vi "Autonomous Independent.vi"() -> ()   [LabVIEW 2016]
doc: "This VI is called when autonomous begins, and will automatically be terminated when autonomous ends. You can carry out timed or sensor driven robot movement independently without needing to return to the caller."
uses:
  2_8_17/Auto_Action.ctl
  <vilib>/Rock Robotics/WPI/Solenoid/WPI_SolenoidValue.ctl
  <vilib>/Rock Robotics/Network Tables/NT Read Number.vi
  <vilib>/Rock Robotics/WPI/Ultrasonic/WPI_SonarSRF04DigitalRefNum Registry Get.vi
  <vilib>/Rock Robotics/WPI/Ultrasonic/WPI_SonarSRF04DigitalGetRange.vi
panel:
  in  "Value":T1=enum."Forward"
  out "Auto Mode":dbl=3.0
  in  "Auton_Modes":T3(array[cluster])=[{"Actions"=[{"Effort"=0.55, "Duration"=3.5, "Action"=enum."Nothing"}, {"Effort"=0.0, "Duration"=0.0, "Action"=enum."Nothing"}]}, {"Actions"=[{"Effort"=0.0, "Duration"=1.0, "Action"=enum."Nothing"}, {"Effort"=0.75, "Duration"=5.0, "Action"=enum."Nothing"}, {"Effort"=0.0, "Duration"=1.0, "Action"=enum."Nothing"}]}, {"Actions"=[{"Effort"=1.0, "Duration"=3.0, "Action"=enum."Nothing"}, {"Effort"=0.0, "Duration"=1.0, "Action"=enum."Nothing"}, {"Effort"=0.75, "Duration"=3.5, "Action"=enum."Nothing"}, {"Effort"=0.0, "Duration"=1.0, "Action"=enum."Nothing"}]}, {"Actions"=[{"Effort"=0.0, "Duration"=0.5, "Action"=enum."Nothing"}, {"Effort"=0.8, "Duration"=5.28, "Action"=enum."Nothing"}, {"Effort"=0.0, "Duration"=1.0, "Action"=enum."Nothing"}, {"Effort"=-0.8, "Duration"=1.8, "Action"=enum."Nothing"}, {"Effort"=0.0, "Duration"=0.1, "Action"=enum."Nothing"}, {"Effort"=0.8, "Duration"=1.75, "Action"=enum."Nothing"}, {"Effort"=0.0, "Duration"=0.5, "Action"=enum."Nothing"}, {"Effort"=0.0, "Duration"=4.0, "Action"=enum."Nothing"}]}, {"Actions"=[{"Effort"=0.0, "Duration"=0.0, "Action"=enum."Nothing"}, {"Effort"=1.0, "Duration"=0.1, "Action"=enum."Nothing"}, {"Effort"=0.0, "Duration"=0.1, "Action"=enum."Nothing"}, {"Effort"=1.0, "Duration"=3.0, "Action"=enum."Nothing"}]}, {"Actions"=[{"Effort"=0.0, "Duration"=0.0, "Action"=enum."Nothing"}, {"Effort"=1.0, "Duration"=0.1, "Action"=enum."Nothing"}, {"Effort"=0.0, "Duration"=0.1, "Action"=enum."Nothing"}, {"Effort"=1.0, "Duration"=3.0, "Action"=enum."Nothing"}]}, {"Actions"=[{"Effort"=0.55, "Duration"=4.0, "Action"=enum."Nothing"}, {"Effort"=0.0, "Duration"=1.0, "Action"=enum."Nothing"}, {"Effort"=-0.5, "Duration"=0.6, "Action"=enum."Nothing"}, {"Effort"=0.75, "Duration"=1.0, "Action"=enum."Nothing"}, {"Effort"=0.0, "Duration"=1.0, "Action"=enum."Nothing"}, {"Effort"=0.75, "Duration"=3.0, "Action"=enum."Nothing"}]}, {"Actions"=[{"Effort"=0.0, "Duration"=0.5, "Action"=enum."Nothing"}, {"Effort"=0.55, "Duration"=4.25, "Action"=enum."Nothing"}, {"Effort"=0.0, "Duration"=0.0, "Action"=enum."Nothing"}, {"Effort"=0.0, "Duration"=0.3, "Action"=enum."Nothing"}, {"Effort"=0.9, "Duration"=2.0, "Action"=enum."Nothing"}]}, {"Actions"=[{"Effort"=0.0, "Duration"=0.0, "Action"=enum."Nothing"}]}]
  # "Nothing"
  # "Boiler Side Gear"
  # "Middle Gear"
  # "Farside Gear"
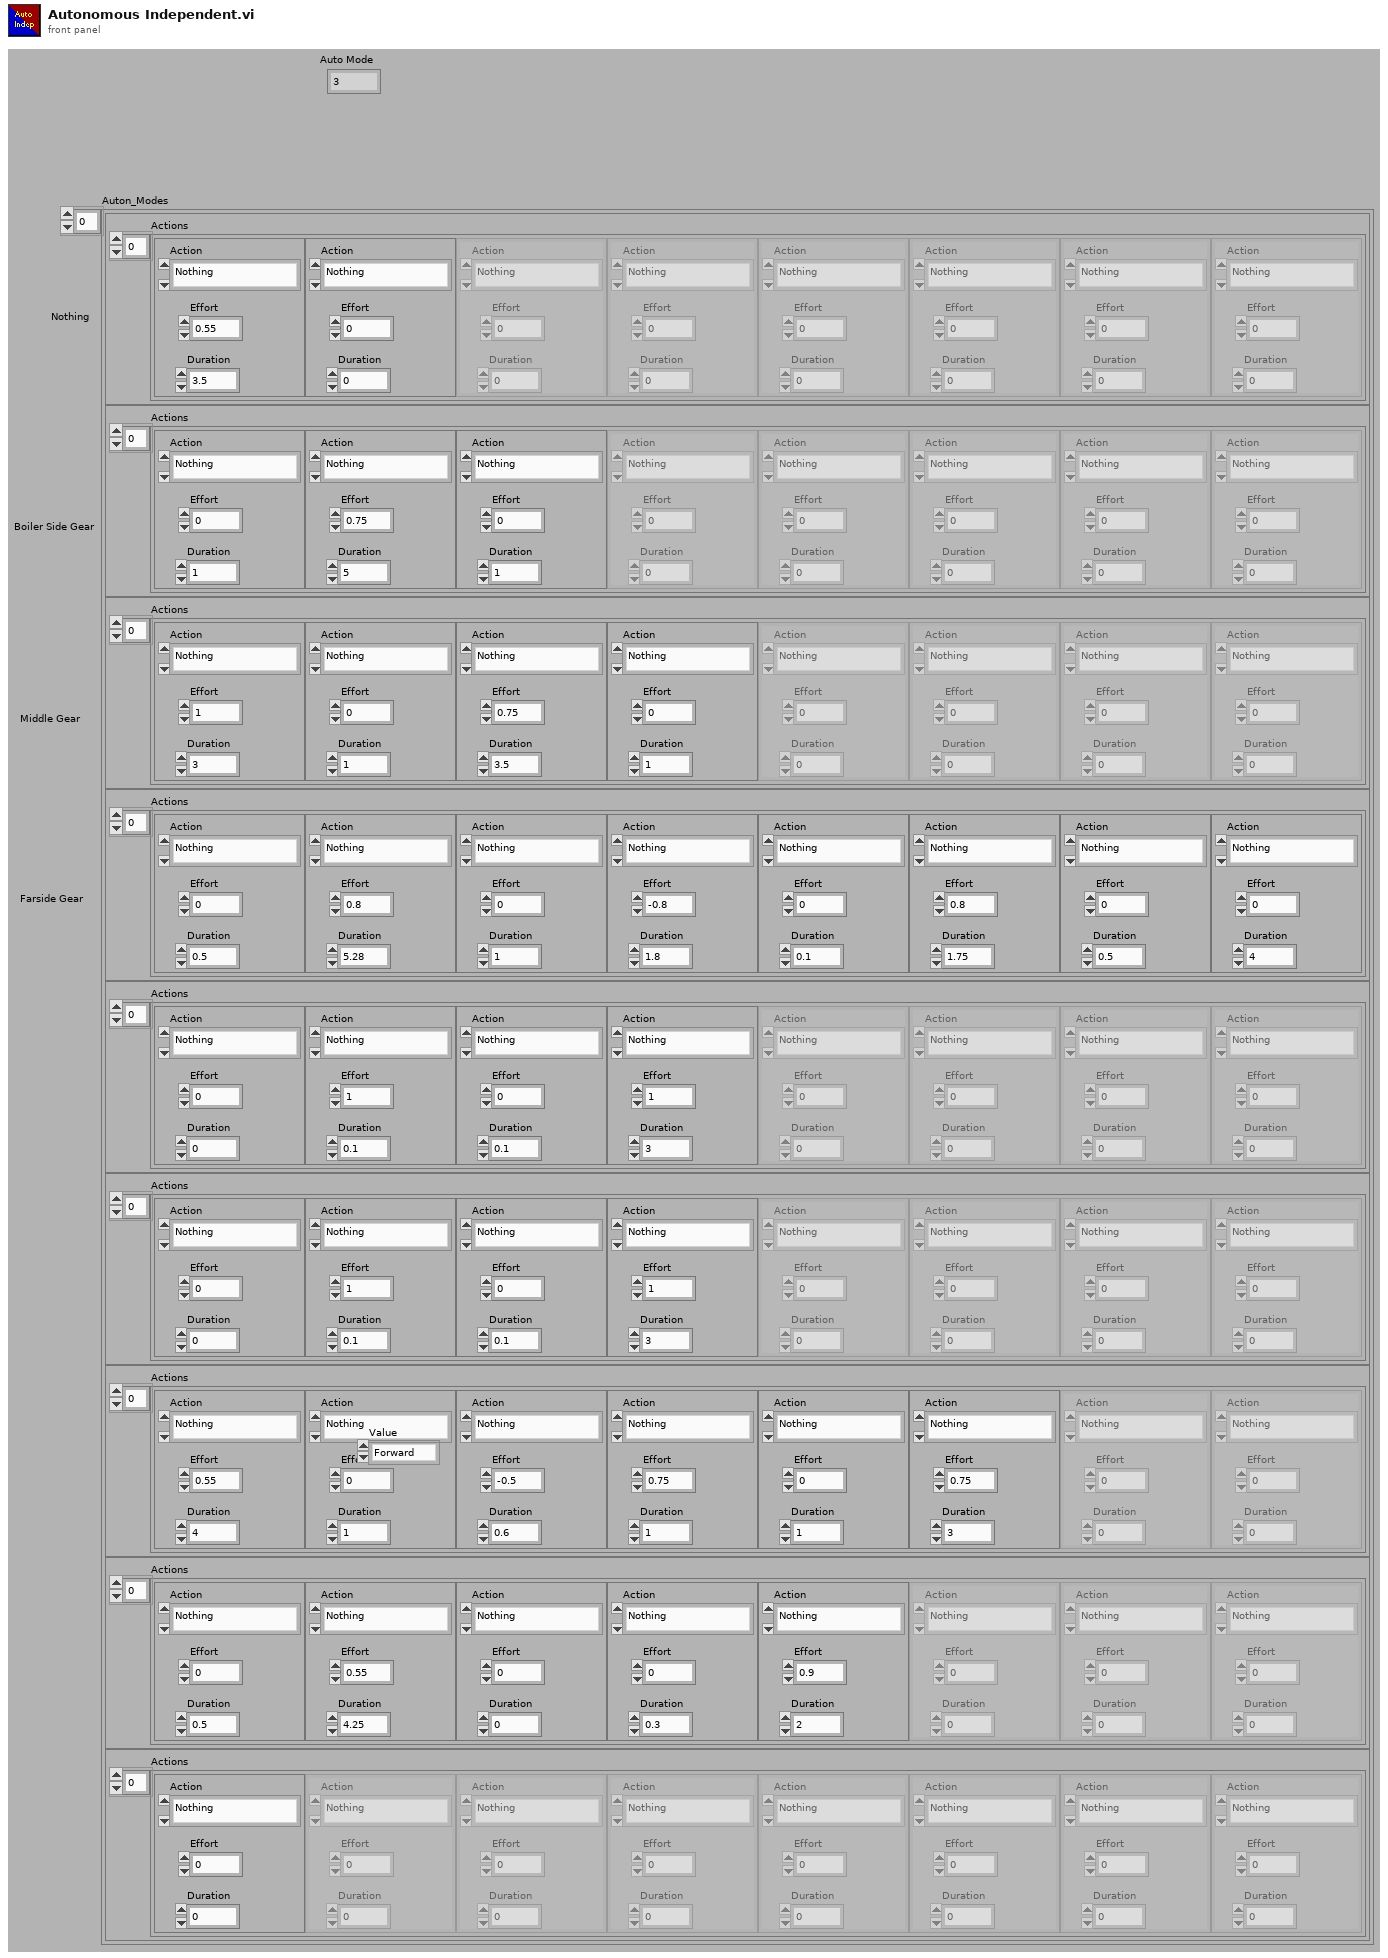
[diagram p1: front panel]
types:
  T1 = typedef "WPI_SolenoidValue.ctl" = enum16{"Off", "On", "Forward", "Reverse"}
  T2 = typedef "Auto_Action.ctl" = enum16{"Nothing", "Drive", "Vision Correction", "Turn", "Gear0", "Gear1", "Climb", "Intake", "Index", "Shoot", "Test", "Drive Encoder Reset", "Gyro Reset"}
  T3 = cluster{"Actions":cluster{"Effort":dbl, "Duration":dbl, "Action":T2}[]}[]
  T4 = cluster{"Actions":cluster{"Effort":dbl, "Duration":dbl, "Action":T2}[]}
  T5 = cluster{"Effort":dbl, "Duration":dbl, "Action":T2}[]
  T6 = typedef "WPI_MotorControlDeviceRef.ctl" = cluster{"DeviceStatus":errorcluster, "Type":T7, "PWM":cluster{"PWM Channel":T8, "DeadBand":T9}, "CAN":cluster{"Device Number":u8, "SetOutput VI Ref":variant, "GetOutput VI Ref":variant, "Enable VI Ref":variant, "Disable VI Ref":variant, "Data":variant}, "Invert":bool}
  T7 = typedef "WPI_MotorControlType.ctl" = enum16{"PWM", "CAN"}
  T8 = typedef "FPGA_DIOPWMChannel.ctl" = enum8{"PWM 0", "PWM 1", "PWM 2", "PWM 3", "PWM 4", "PWM 5", "PWM 6", "PWM 7", "PWM 8", "PWM 9", "PWM MXP 0", "PWM MXP 1", "PWM MXP 2", "PWM MXP 3", "PWM MXP 4", "PWM MXP 5", "PWM MXP 6", "PWM MXP 7", "PWM MXP 8", "PWM MXP 9", "Invalid"}
  T9 = typedef "WPI_PWMDeadband.ctl" = cluster{"Name":string, "maxPositivePwm":i32, "minPositivePwm":i32, "centerPwm":i32, "maxNegativePwm":i32, "minNegativePwm":i32, "angularRange":u16}
  T10 = typedef "WPI_UltrasonicDeviceRef.ctl" = cluster{"DevStatus":errorcluster, "Ping Channel":T11, "Echo Channel":T11, "CntIndex":T12}
  T11 = typedef "FPGA_DIOChannel.ctl" = enum8{"DIO 0", "DIO 1", "DIO 2", "DIO 3", "DIO 4", "DIO 5", "DIO 6", "DIO 7", "DIO 8", "DIO 9", "DIO MXP 0", "DIO MXP 1", "DIO MXP 2", "DIO MXP 3", "DIO MXP 4", "DIO MXP 5", "DIO MXP 6", "DIO MXP 7", "DIO MXP 8", "DIO MXP 9", "DIO MXP 10", "DIO MXP 11", "DIO MXP 12", "DIO MXP 13", "DIO MXP 14", "DIO MXP 15", "SPI Port CS1", "SPI Port CS2", "SPI Port CS3", "SPI Port MISO", "SPI Port MOSI", "Invalid"}
  T12 = typedef "FPGA_CounterCtrSystemIndex.ctl" = enum8{"Ctr 0", "Ctr 1", "Ctr 2", "Ctr 3", "Ctr 4", "Ctr 5", "Ctr 6", "Ctr 7", "Invalid"}
  T13 = typedef "WPI_GyroDevRef.ctl" = cluster{"DevStatus":errorcluster, "Analog Channel":T14, "Offset":dbl, "Gain (VoltsPerDegree/Second)":dbl, "Gyro Type":enum16{"Analog", "XRS450"}, "Handle":i32, "SPI Bus":T15, "Device Found":bool, "Sample Rate":dbl, "Calibrate On Open":bool}
  T14 = typedef "FPGA_AIChannel.ctl" = enum8{"AI 0", "AI 1", "AI 2", "AI 3", "AI MXP 0", "AI MXP 1", "AI MXP 2", "AI MXP 3", "Invalid"}
  T15 = typedef "spi_bus.ctl" = enum16{"SPI On-Board, CS0", "SPI On-Board, CS1", "SPI On-Board, CS2", "SPI On-Board, CS3", "SPI MXP", "Invalid"}
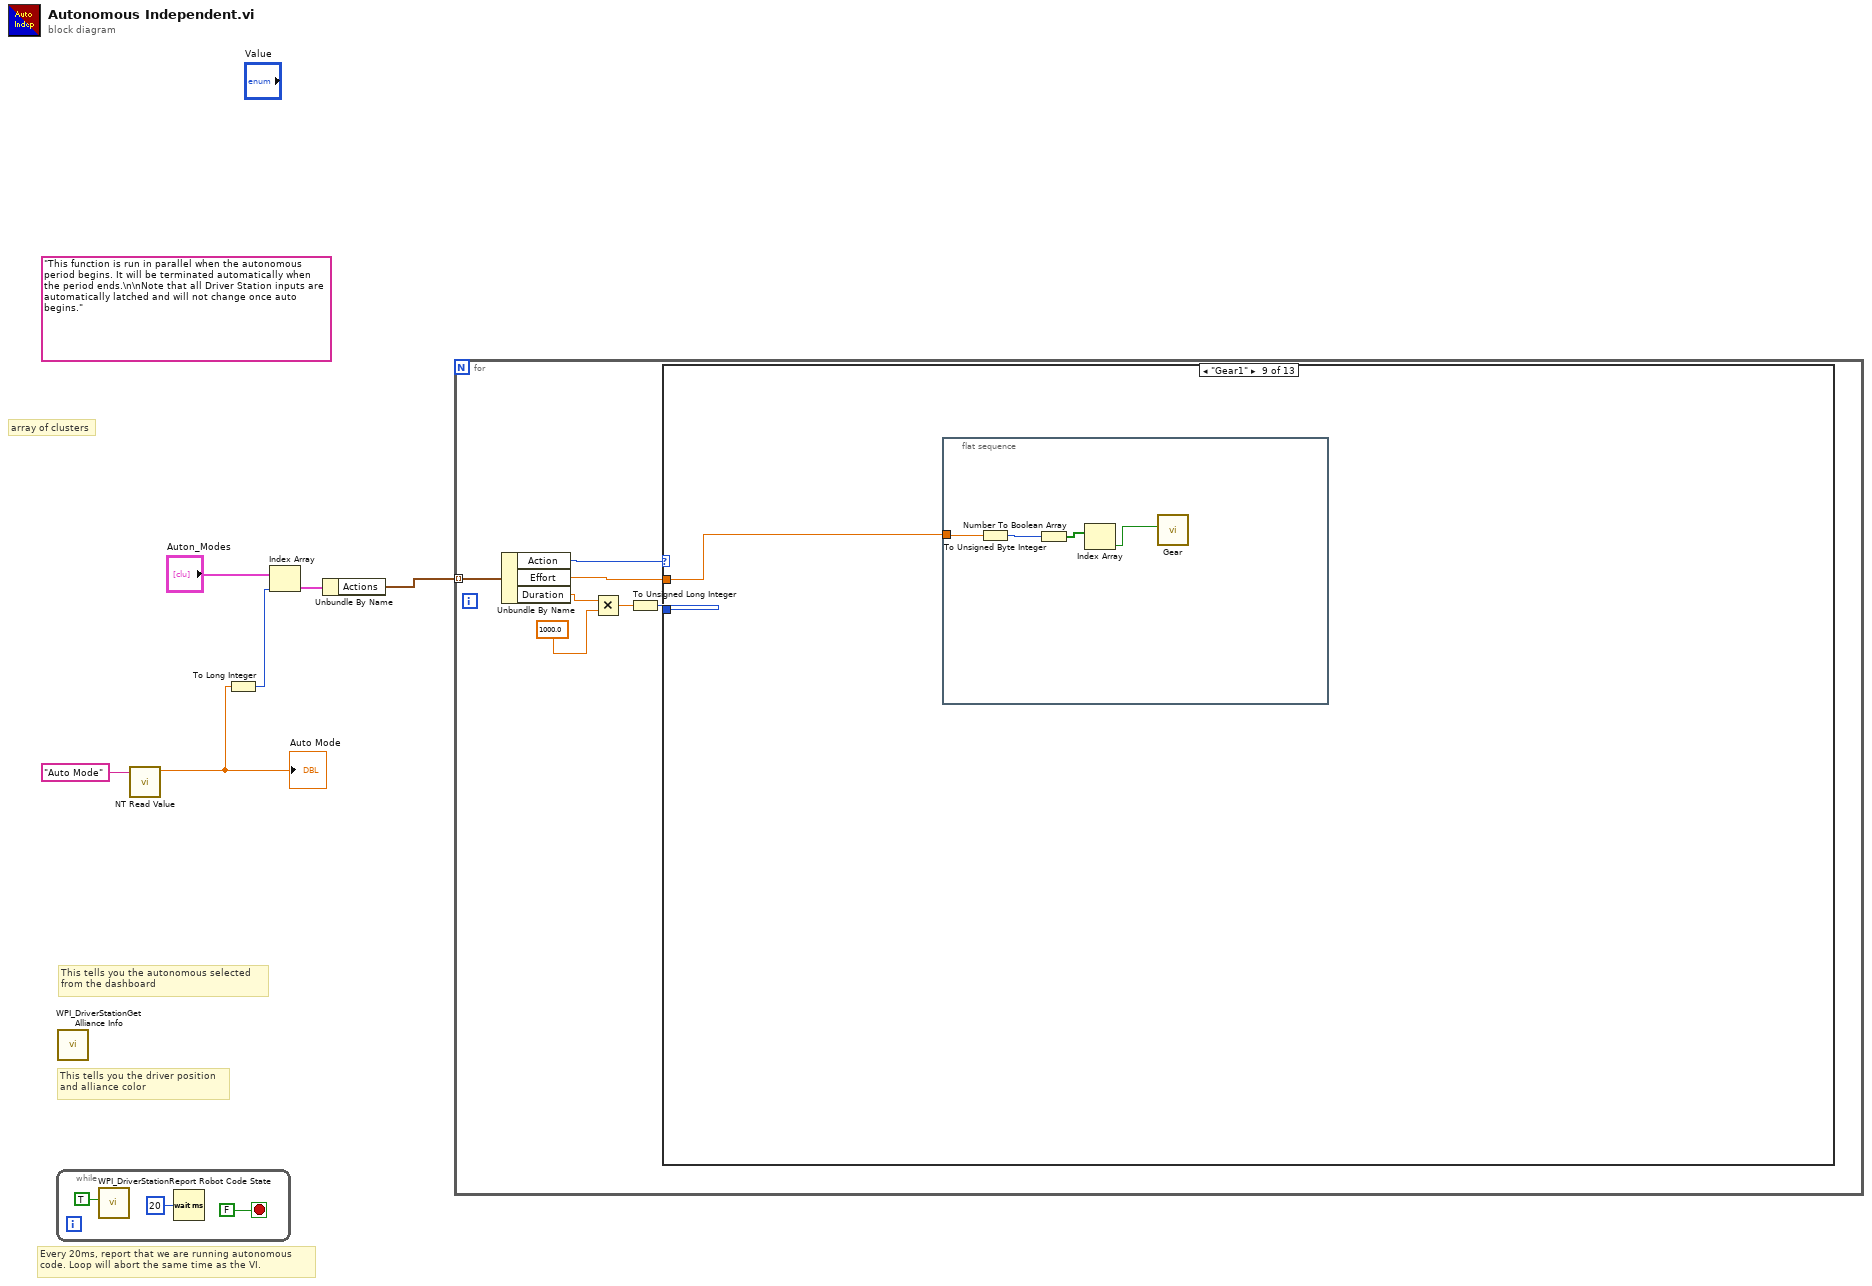
[diagram p0: block diagram]
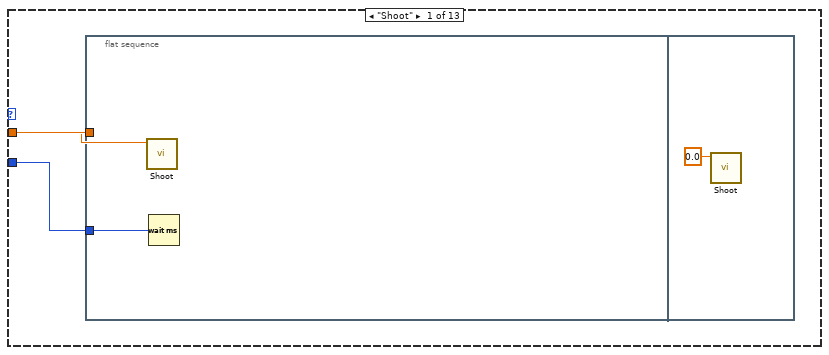
[diagram p2: hidden frame]
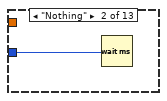
[diagram p3: hidden frame]
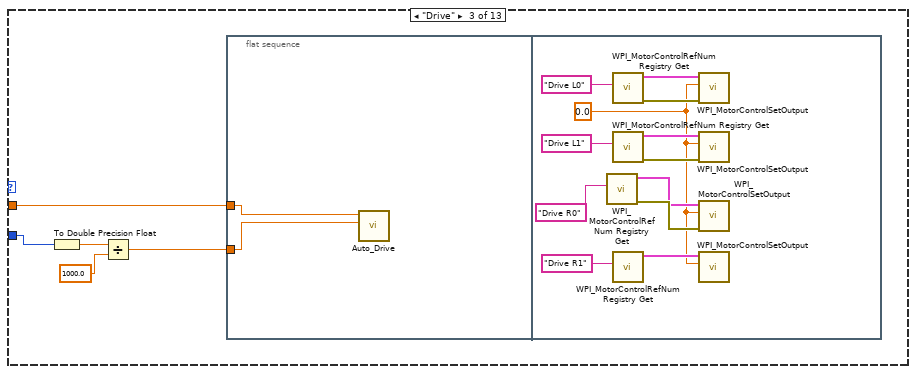
[diagram p4: hidden frame]
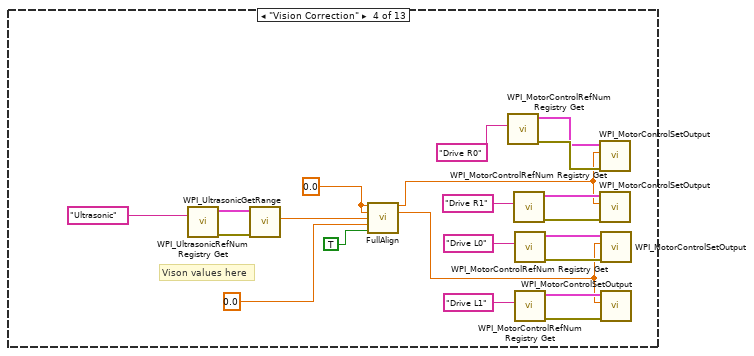
[diagram p5: hidden frame]
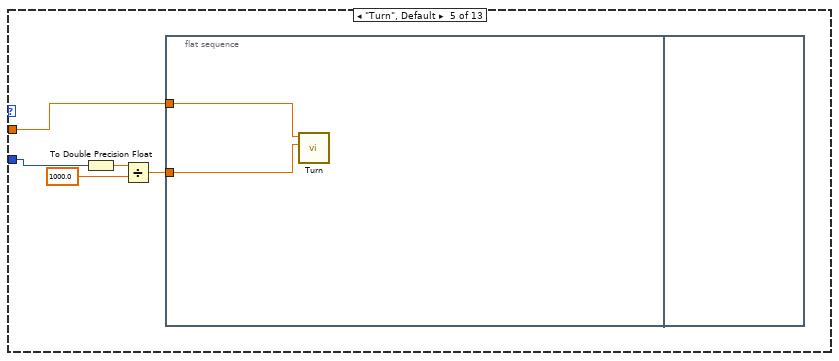
[diagram p6: hidden frame]
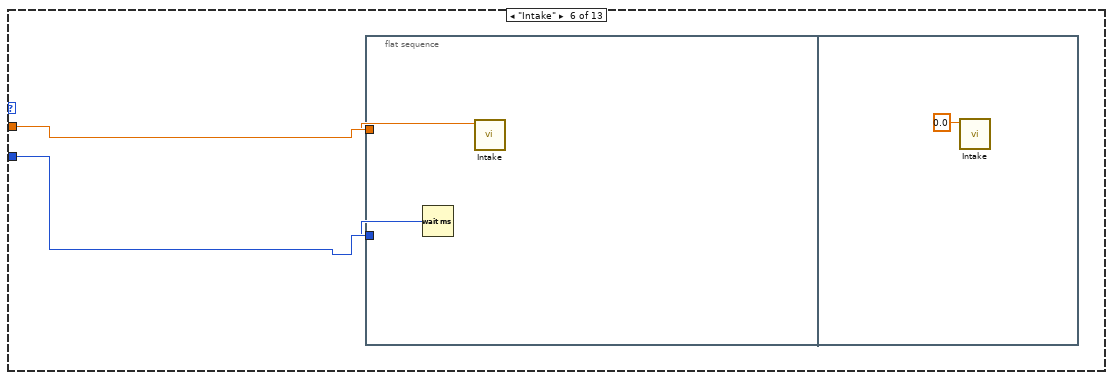
[diagram p7: hidden frame]
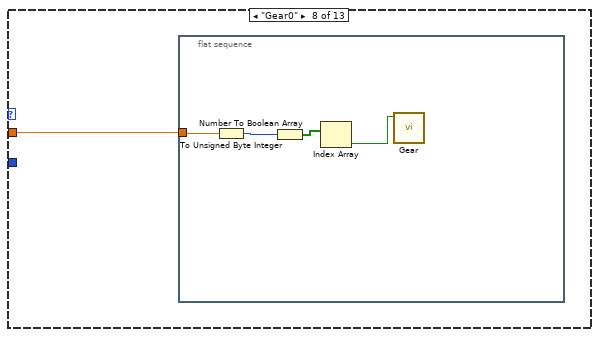
[diagram p9: hidden frame]
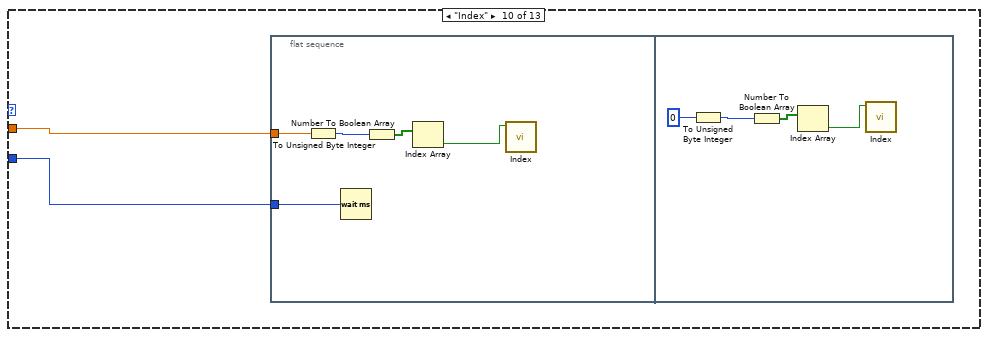
[diagram p10: hidden frame]
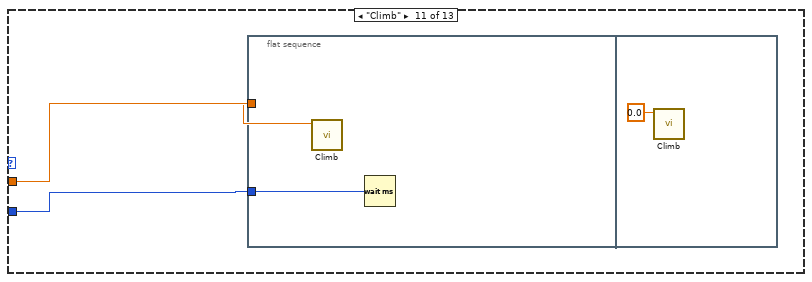
[diagram p11: hidden frame]
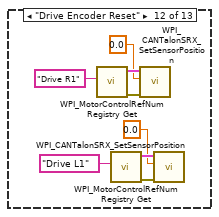
[diagram p12: hidden frame]
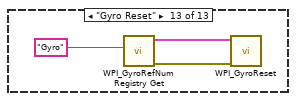
[diagram p13: hidden frame]
diagram:
  (unwired) "This function is run in parallel when the autonomous period begins. It will be terminated automatically when the period ends.\n\nNote that all Driver Station inputs are automatically latched and will not change once auto begins."
  # "This tells you the autonomous selected\nfrom the dashboard"
  # "array of clusters"
  # "Every 20ms, report that we are running autonomous\ncode. Loop will abort the same time as the VI."
  # "This tells you the driver position\nand alliance color"
  n1 = while {
    stop <- FALSE stop-if-true
    n2 = call <vilib>:"WPI_DriverStationReport Robot Code State.vi"("Autonomous"=TRUE) -> ()  [unwired: 10 in, 1 out]
    n3 = Wait (ms)(milliseconds to wait=u32 20) -> ()  [unwired: 1 out]
  }
  n4 = call <vilib>:"WPI_DriverStationGet Alliance Info.vi"() -> ()  [unwired: 12 out]
  n5 = call-poly <vilib>:"NT Read Value.vi"("Name"="Auto Mode") -> ("Numeric"=w1:dbl)  [unwired: 9 in, 1 out]
  "Auto Mode" <- w1
  n6 = To Long Integer(number=w1) -> (32bit integer=w3:i32)
  n7 = Index Array(array="Auton_Modes", index=w3) -> (element=w5:T4)
  n8 = Unbundle By Name(w5) -> ("Actions"=w6:T5)
  n9 = for {
    tunnel: w6 -> [w16] mode=indexing
    n10 = Unbundle By Name(w16) -> ("Action"=w15:T2, "Effort"=w14:dbl, "Duration"=w13:dbl)
    n11 = Multiply(x=w13, y=1000.0) -> (x*y=w11:dbl)
    n12 = To Unsigned Long Integer(number=w11) -> (unsigned 32bit integer=w10:u32)
    n13 = case shown="\"Gear1\"" w15 {
      tunnel: w14 -> [w18 _ w27 _ w67 w71 _ w75 w80 w85 w97 _ _]
      tunnel: w10 -> [w17 w22 w26 _ w66 w70 _ _ _ w86 w96 _ _]
      frame "Shoot" {
        n14 = flat-sequence {
          tunnel: w18 -> [w20]
          tunnel: w17 -> [w19]
          frame #0 {
            n15 = call "Shoot.vi"("Effort"=w20) -> ()  [unwired: 11 in]
            n16 = Wait (ms)(milliseconds to wait=w19) -> ()  [unwired: 1 out]
          }
          frame #1 {
            n17 = call "Shoot.vi"("Effort"=0.0) -> ()  [unwired: 11 in]
          }
        }
      }
      frame "Nothing" {
        n18 = Wait (ms)(milliseconds to wait=w22) -> ()  [unwired: 1 out]
      }
      frame "Drive" {
        n19 = To Double Precision Float(number=w26) -> (double precision float=w25:dbl)
        n20 = Divide(x=w25, y=1000.0) -> (x/y=w23:dbl)
        n21 = flat-sequence {
          tunnel: w27 -> [w29]
          tunnel: w23 -> [w28]
          frame #0 {
            n22 = call "Auto_Drive.vi"("Duration"=w28, "Drive Effort"=w29) -> ()  [unwired: 10 in]
          }
          frame #1 {
            w30 = 0.0 ("Drive L")
            n23 = call <vilib>:"WPI_MotorControlRefNum Registry Get.vi"("refnum name"="Drive R0") -> ("error out"=w35:errorcluster, "MotorControlDevRef"=w31:T6)  [unwired: 9 in]
            n24 = call <vilib>:"WPI_MotorControlRefNum Registry Get.vi"("refnum name"="Drive L0") -> ("error out"=w36:errorcluster, "MotorControlDevRef"=w37:T6)  [unwired: 9 in]
            n25 = call <vilib>:"WPI_MotorControlRefNum Registry Get.vi"("refnum name"="Drive L1") -> ("error out"=w40:errorcluster, "MotorControlDevRef"=w39:T6)  [unwired: 9 in]
            n26 = call <vilib>:"WPI_MotorControlRefNum Registry Get.vi"("refnum name"="Drive R1") -> ("MotorControlDevRef"=w33:T6)  [unwired: 9 in, 1 out]
            n27 = call <vilib>:"WPI_MotorControlSetOutput.vi"("error in (no error)"=w36, "Output"=w30, "MotorControlDevRef"=w37) -> ()  [unwired: 6 in, 3 out]
            n28 = call <vilib>:"WPI_MotorControlSetOutput.vi"("error in (no error)"=w40, "Output"=w30, "MotorControlDevRef"=w39) -> ()  [unwired: 6 in, 3 out]
            n29 = call <vilib>:"WPI_MotorControlSetOutput.vi"("error in (no error)"=w35, "Output"=w30, "MotorControlDevRef"=w31) -> ()  [unwired: 6 in, 3 out]
            n30 = call <vilib>:"WPI_MotorControlSetOutput.vi"("Output"=w30, "MotorControlDevRef"=w33) -> ()  [unwired: 7 in, 3 out]
          }
        }
      }
      frame "Vision Correction" {
        w62 = 0.0
        # "Vison values here"
        n31 = call-poly <vilib>:"WPI_UltrasonicRefNum Registry Get.vi"("refnum name"="Ultrasonic") -> ("error out"=w61:errorcluster, "SonarSRF04DevRef"=w60:T10)  [unwired: 9 in]
        n32 = call-poly <vilib>:"WPI_UltrasonicGetRange.vi"("error in (no error)"=w61, "SonarSRF04DevRef"=w60) -> ("Distance"=w59:dbl)  [unwired: 7 in, 2 out]
        n33 = call "FullAlign.vi"("Joystick 0"=w62, "Joystick 1"=w62, "Distance"=w59, "Angle"=0.0, "Button"=TRUE) -> ("Right Motor"=w44:dbl, "Left Motor"=w43:dbl)  [unwired: 6 in, 3 out]
        n34 = call <vilib>:"WPI_MotorControlRefNum Registry Get.vi"("refnum name"="Drive R0") -> ("error out"=w50:errorcluster, "MotorControlDevRef"=w46:T6)  [unwired: 9 in]
        n35 = call <vilib>:"WPI_MotorControlRefNum Registry Get.vi"("refnum name"="Drive R1") -> ("error out"=w45:errorcluster, "MotorControlDevRef"=w48:T6)  [unwired: 9 in]
        n36 = call <vilib>:"WPI_MotorControlRefNum Registry Get.vi"("refnum name"="Drive L0") -> ("error out"=w51:errorcluster, "MotorControlDevRef"=w52:T6)  [unwired: 9 in]
        n37 = call <vilib>:"WPI_MotorControlRefNum Registry Get.vi"("refnum name"="Drive L1") -> ("error out"=w55:errorcluster, "MotorControlDevRef"=w54:T6)  [unwired: 9 in]
        n38 = call <vilib>:"WPI_MotorControlSetOutput.vi"("error in (no error)"=w50, "Output"=w44, "MotorControlDevRef"=w46) -> ()  [unwired: 6 in, 3 out]
        n39 = call <vilib>:"WPI_MotorControlSetOutput.vi"("error in (no error)"=w45, "Output"=w44, "MotorControlDevRef"=w48) -> ()  [unwired: 6 in, 3 out]
        n40 = call <vilib>:"WPI_MotorControlSetOutput.vi"("error in (no error)"=w51, "Output"=w43, "MotorControlDevRef"=w52) -> ()  [unwired: 6 in, 3 out]
        n41 = call <vilib>:"WPI_MotorControlSetOutput.vi"("error in (no error)"=w55, "Output"=w43, "MotorControlDevRef"=w54) -> ()  [unwired: 6 in, 3 out]
      }
      frame "Turn", Default {
        n42 = To Double Precision Float(number=w66) -> (double precision float=w65:dbl)
        n43 = Divide(x=w65, y=1000.0) -> (x/y=w63:dbl)
        n44 = flat-sequence {
          tunnel: w67 -> [w69]
          tunnel: w63 -> [w68]
          frame #0 {
            n45 = call "Turn.vi"("Angle"=w68, "Effort"=w69) -> ()  [unwired: 10 in]
          }
          frame #1 {
          }
        }
      }
      frame "Intake" {
        n46 = flat-sequence {
          tunnel: w71 -> [w73]
          tunnel: w70 -> [w72]
          frame #0 {
            n47 = Wait (ms)(milliseconds to wait=w72) -> ()  [unwired: 1 out]
            n48 = call "Intake.vi"("Effort"=w73) -> ()  [unwired: 11 in]
          }
          frame #1 {
            n49 = call "Intake.vi"("Effort"=0.0) -> ()  [unwired: 11 in]
          }
        }
      }
      frame "Test" {
      }
      frame "Gear0" {
        n50 = flat-sequence {
          tunnel: w75 -> [w79]
          frame #0 {
            n51 = To Unsigned Byte Integer(number=w79) -> (unsigned 8bit integer=w78:u8)
            n52 = Number To Boolean Array(number=w78) -> (Boolean array=w77:bool[])
            n53 = Index Array(array=w77) -> (element=w76:bool)  [unwired: 1 in]
            n54 = call "Gear.vi"("Gear0?"=w76) -> ()  [unwired: 11 in]
          }
        }
      }
      frame "Gear1" {
        n55 = flat-sequence {
          tunnel: w80 -> [w84]
          frame #0 {
            n56 = To Unsigned Byte Integer(number=w84) -> (unsigned 8bit integer=w83:u8)
            n57 = Number To Boolean Array(number=w83) -> (Boolean array=w82:bool[])
            n58 = Index Array(array=w82) -> (element=w81:bool)  [unwired: 1 in]
            n59 = call "Gear.vi"("Gear1?"=w81) -> ()  [unwired: 11 in]
          }
        }
      }
      frame "Index" {
        n60 = flat-sequence {
          tunnel: w86 -> [w88]
          tunnel: w85 -> [w87]
          frame #0 {
            n61 = To Unsigned Byte Integer(number=w87) -> (unsigned 8bit integer=w91:u8)
            n62 = Wait (ms)(milliseconds to wait=w88) -> ()  [unwired: 1 out]
            n63 = Number To Boolean Array(number=w91) -> (Boolean array=w90:bool[])
            n64 = Index Array(array=w90) -> (element=w89:bool)  [unwired: 1 in]
            n65 = call "Index.vi"("Index?"=w89) -> ()  [unwired: 11 in]
          }
          frame #1 {
            n66 = To Unsigned Byte Integer(number=u8 0) -> (unsigned 8bit integer=w94:u8)
            n67 = Number To Boolean Array(number=w94) -> (Boolean array=w95:bool[])
            n68 = Index Array(array=w95) -> (element=w92:bool)  [unwired: 1 in]
            n69 = call "Index.vi"("Index?"=w92) -> ()  [unwired: 11 in]
          }
        }
      }
      frame "Climb" {
        n70 = flat-sequence {
          tunnel: w97 -> [w99]
          tunnel: w96 -> [w98]
          frame #0 {
            n71 = call "Climb.vi"("Effort"=w99) -> ()  [unwired: 11 in]
            n72 = Wait (ms)(milliseconds to wait=w98) -> ()  [unwired: 1 out]
          }
          frame #1 {
            n73 = call "Climb.vi"("Effort"=0.0) -> ()  [unwired: 11 in]
          }
        }
      }
      frame "Drive Encoder Reset" {
        n74 = call <vilib>:"WPI_MotorControlRefNum Registry Get.vi"("refnum name"="Drive R1") -> ("error out"=w103:errorcluster, "MotorControlDevRef"=w102:T6)  [unwired: 9 in]
        n75 = call <vilib>:"WPI_MotorControlRefNum Registry Get.vi"("refnum name"="Drive L1") -> ("error out"=w105:errorcluster, "MotorControlDevRef"=w106:T6)  [unwired: 9 in]
        n76 = call <vilib>:"WPI_CANTalonSRX_SetSensorPosition.vi"("error in (no error)"=w103, "New Sensor Position"=0.0, "CAN Talon SRX Ref"=w102) -> ()  [unwired: 7 in, 2 out]
        n77 = call <vilib>:"WPI_CANTalonSRX_SetSensorPosition.vi"("error in (no error)"=w105, "New Sensor Position"=0.0, "CAN Talon SRX Ref"=w106) -> ()  [unwired: 7 in, 2 out]
      }
      frame "Gyro Reset" {
        n78 = call <vilib>:"WPI_GyroRefNum Registry Get.vi"("refnum name"="Gyro") -> ("error out"=w110:errorcluster, "GyroDevRef"=w111:T13)  [unwired: 9 in]
        n79 = call <vilib>:"WPI_GyroReset.vi"("error in"=w110, "GyroDevRef"=w111) -> ()  [unwired: 8 in, 2 out]
      }
    }
  }
